vi "Shut_Down_EnFlo_Lab.vi"   [LabVIEW 2013]
uses:
  ADAM Client/Sub VIs/ADAM Controls/Function_ADAM.ctl
  ADAM Client/Sub VIs/ADAM Controls/Channel_State.ctl
  ADAM_Global.vi
types:
  T1 = typedef "Ch_description_ADAM.ctl" = cluster{"Ch Name":string, "Type":T2, "Function":T3, "Ch State":T4, "Calibration type":T5, "A":dbl, "B":dbl, "C":dbl, "D":dbl, "Comments":string, "Address":T6, "String":string, "Duty":u16}
  T2 = typedef "Module_type_ADAM.ctl" = string
  T3 = typedef "Function_ADAM.ctl" = enum16{"Analogue Input", "Digital Input", "Event counter", "Event rate", "Analogue Output", "Digital Output", "Relay Output"}
  T4 = typedef "Channel_State.ctl" = enum16{"On", "Off", "Always On", "Always Off"}
  T5 = typedef "Calib_type_ADAM.ctl" = enum16{"Raw", "Bx + A", "Cx^2 + Bx + A", "Dx^3 + Cx^2 + Bx + A", "In Band", "Hi-Tec Q", "Hi-Tec M_dot", "Text"}
  T6 = typedef "Address.ctl" = cluster{"Main":i32, "Ch.":i32, "Sub":i32, "Port Name":string}
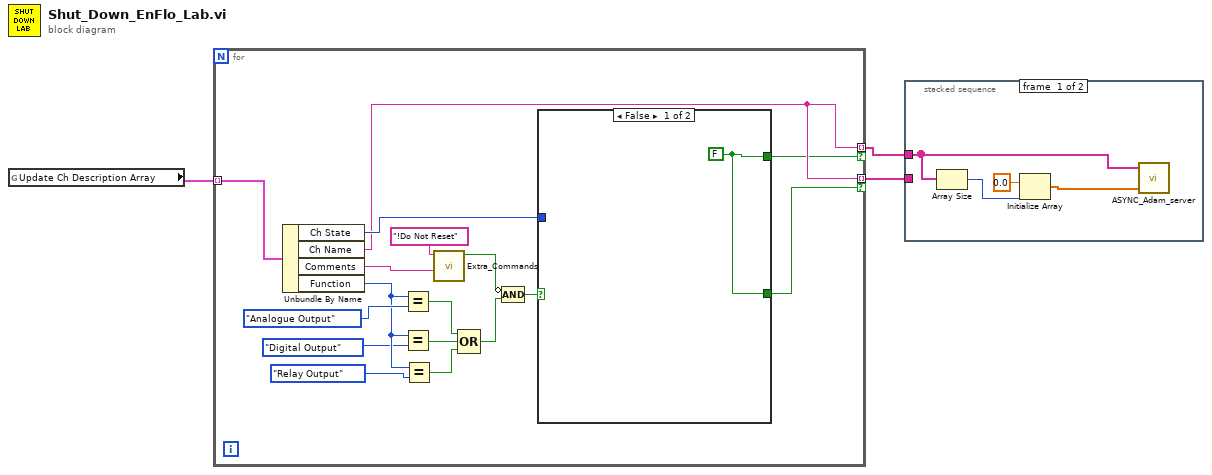
[diagram p0: block diagram]
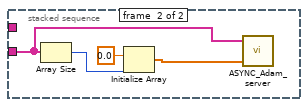
[diagram p2: hidden frame]
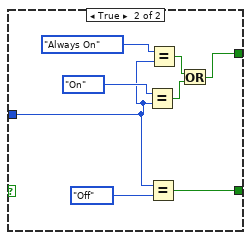
[diagram p3: hidden frame]
diagram:
  n1 = global read "ADAM_Global.vi" "Update Ch Description Array"() -> (w3:T1[])
  n2 = for {
    tunnel: w3 -> [w20] mode=indexing
    tunnel: [w6] -> w2 mode=indexing if=w5
    tunnel: [w6] -> w1 mode=indexing if=w4
    n3 = Unbundle By Name(w20) -> ("Ch State"=w7:T4, "Ch Name"=w6:string, "Comments"=w11:string, "Function"=w18:T3)
    n4 = Equal?(x=w18, y=Function_ADAM."Analogue Output" ("Function")) -> (x = y?=w15:bool)
    n5 = Equal?(x=w18, y=Function_ADAM."Digital Output" ("Function")) -> (x = y?=w14:bool)
    n6 = Equal?(x=w18, y=Function_ADAM."Relay Output" ("Function")) -> (x = y?=w13:bool)
    n7 = call "Extra_Commands.vi"("String to Search"=w11, "Command"="!Do Not Reset" ("String to match")) -> ("Command Found"=w9:bool)  [unwired: 1 in, 4 out]
    n8 = Compound Arithmetic op=OR(w15, w14, w13) -> (w10:bool)
    n9 = Compound Arithmetic op=AND(invert w9, w10) -> (w8:bool)
    n10 = case shown="False" w8 {
      tunnel: w7 -> [_ w24]
      tunnel: [w21 w23] -> w5
      tunnel: [w21 w22] -> w4
      frame False {
        w21 = FALSE
      }
      frame True {
        n11 = Equal?(x=Channel_State."On" ("Ch State"), y=w24) -> (x = y?=w26:bool)
        n12 = Equal?(x=w24, y=Channel_State."Off" ("Ch State")) -> (x = y?=w22:bool)
        n13 = Equal?(x=Channel_State."Always On" ("Ch State"), y=w24) -> (x = y?=w27:bool)
        n14 = Or(x=w27, y=w26) -> (x .or. y?=w23:bool)
      }
    }
  }
  n15 = stacked-sequence {
    tunnel: w2 -> [w30 _]
    tunnel: w1 -> [_ w34]
    frame #0 {
      n16 = Array Size(array=w30) -> (size(s)=w32:i32)
      n17 = Initialize Array(0.0 ("element"), w32) -> (w31:dbl[])
      n18 = call "ASYNC_Adam_server.vi"("Values"=w31, "Channel Names"=w30) -> ()  [unwired: 1 in, 3 out]
    }
    frame #1 {
      n19 = Array Size(array=w34) -> (size(s)=w36:i32)
      n20 = Initialize Array(0.0 ("element"), w36) -> (w35:dbl[])
      n21 = call "ASYNC_Adam_server.vi"("Values"=w35, "Channel Names"=w34) -> ()  [unwired: 1 in, 3 out]
    }
  }
